vi "12.2-4 FindCircles.vi"() -> ()   [LabVIEW 2016]
doc: "This example shows how to use the Edge Tool in NI Vision. The Edge Tool finds edges (or sharp transitions in the pixels values) along a given line or ROI profile. The Edge Tool is a precursor function to many of the gauging and inspection tasks. For example, the location of the edges found along a line profile across an object can interpreted as the boundaries of the object whose dimensions have to be measured for a gauging application or the presence of a crack in the surface of an object for an inspection application."
uses:
  <vilib>/vision/NI_Vision_Development_Module.lvlib
panel:
  out "Nb Circles":i32
  out "Circles Data":T1(array[cluster])
  in  "ImgTab":enum32{"Source Image", "Results"}(tab)
  out "Src":T2(plugin-control)
  out "Dst":T2(plugin-control)
  in  "Max Radius":sgl=34.0 format="%.2f"
  in  "Min Radius":sgl=28.0 format="%.2f"
  in  "Stop":bool
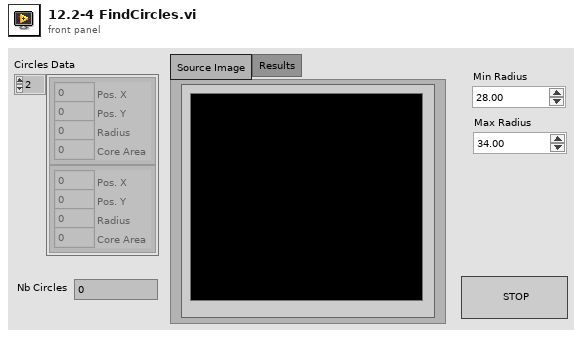
[diagram p1: front panel]
types:
  T1 = cluster{"Pos. X":i32, "Pos. Y":i32, "Radius":i32, "Core Area":i32}[]
  T2 = typedef "IMAQ Image.ctl" = refnum<image>
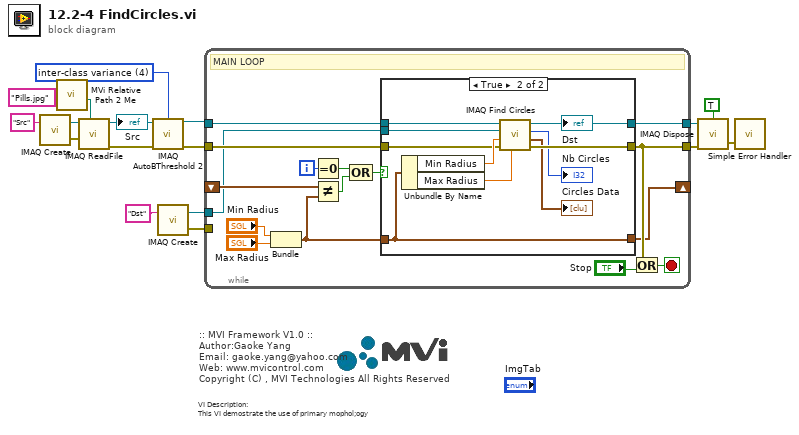
[diagram p0: block diagram]
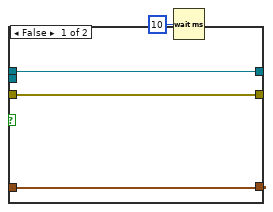
[diagram p2: hidden frame]
diagram:
  w6 = 4 items=["clustering", "entropy", "metric", "moments", "inter-class variance"] ("Method")
  # "VI Description:\nThis VI demostrate the use of primary mophol;ogy"
  # ":: MVI Framework V1.0 ::\nAuthor:Gaoke Yang\nEmail: gaoke.yang@yahoo.com\nWeb: www.mvicontrol.com\nCopyright (C) , MVI Technologies All Rights Reserved"
  n1 = call "IMAQ Create"("Image Name"="Src") -> ("New Image"=w16:T2, "error out"=w15:errorcluster)  [unwired: 4 in]
  n2 = call "MVi Relative Path 2 Me.vi"("Relative Path"="Pills.jpg" ("name or relative path")) -> ("Appended Dir"=w11:path)  [unwired: 5 in, 1 out]
  n3 = call "IMAQ ReadFile"("File Path"=w11, "error in (no error)"=w15, "Image"=w16) -> ("error out"=w5:errorcluster, "Image Out"=w1:T2)  [unwired: 4 in, 3 out]
  "Src" <- w1
  n4 = call "IMAQ AutoBThreshold 2"("Image Src"=w1, "Method (clustering)"=w6, "error in (no error)"=w5) -> ("Image Dst Out"=w2:T2, "error out"=w3:errorcluster)  [unwired: 5 in, 6 out]
  n5 = call "IMAQ Create"("Image Name"="Dst") -> ("New Image"=w8:T2, "error out"=w7:errorcluster)  [unwired: 4 in]
  n6 = while "MAIN LOOP" {
    tunnel: w2 -> [w32]
    tunnel: w3 -> [w33]
    tunnel: [w28] -> w14
    tunnel: [w29] -> w13
    shift-right: [w25] -> _
    shift-left: _ -> [w22]
    tunnel: w8 -> [w20]
    tunnel: w7 -> [_]
    i -> [w27]
    stop <- w30 stop-if-true
    # "MAIN LOOP"
    n7 = Bundle("Min Radius"="Min Radius", "Max Radius"="Max Radius") -> (w23:cluster{"Min Radius":sgl, "Max Radius":sgl})  [unwired: 1 in]
    n8 = Equal To 0?(x=w27) -> (x = 0?=w24:bool)
    n9 = Not Equal?(x=w22, y=w23) -> (x != y?=w21:bool)
    n10 = Compound Arithmetic op=OR(w24, w21) -> (w26:bool)
    n11 = case shown="True" w26 {
      tunnel: w33 -> [w36 w44]
      tunnel: w32 -> [w37 w42]
      tunnel: [w37 w40] -> w29
      tunnel: [w36 w43] -> w28
      tunnel: [w34 w47] -> w25
      tunnel: w23 -> [w34 w47]
      tunnel: w20 -> [_ w41]
      frame False {
        n12 = Wait (ms)(milliseconds to wait=u32 10) -> ()  [unwired: 1 out]
      }
      frame True {
        n13 = Unbundle By Name(w47) -> ("Min Radius"=w45:sgl, "Max Radius"=w46:sgl)
        n14 = call "IMAQ Find Circles"("Max Radius"=w46, "error in (no error)"=w44, "Min Radius"=w45, "Image Dst"=w41, "Image Src"=w42) -> ("error out"=w43:errorcluster, "Circles Data"=→"Circles Data":T1, "Nb Circles"=→"Nb Circles":i32, "Image Dst Out"=w40:T2)  [unwired: 3 in]
        "Dst" <- w40
      }
    }
    n15 = Or(x=w28, y="Stop") -> (x .or. y?=w30:bool)
  }
  n16 = call "IMAQ Dispose"("All Images? (No)"=TRUE, "Image"=w13, "error in (no error)"=w14) -> ("error out"=w10:errorcluster)  [unwired: 3 in]
  n17 = call <vilib>:"Simple Error Handler.vi"("error in (no error)"=w10) -> ()  [unwired: 4 in, 5 out]
